vi "adam-analog-outputs.vi"(0 "VISA Refnum in":refnum<visa-resource-name>, 1 "Chassis Settings":T1, 5 "Current AO States":T2, 7 "Analog Outputs in":T2, 9 "chassis-slot":i32, 11 "error in (no error)":errorcluster, 12 "Last cmd":string, 13 "last ack message":string) -> (4 "VISA Refnum out":refnum<visa-resource-name>, 6 "Analog Outputs out":T2, 8 "cmd output":string, 10 "ack message":string, 14 "cmd aknowledged":bool, 15 "error out":errorcluster)   [LabVIEW 2020]
uses:
  controls/analog-output-cluster.ctl
  controls/adam-5000-serial-settings.ctl
panel:
  out "size(s)":i32
  out "loopwise ack":string
  out "OP Num":string
  out "Data":string
  out "live-cmd":string
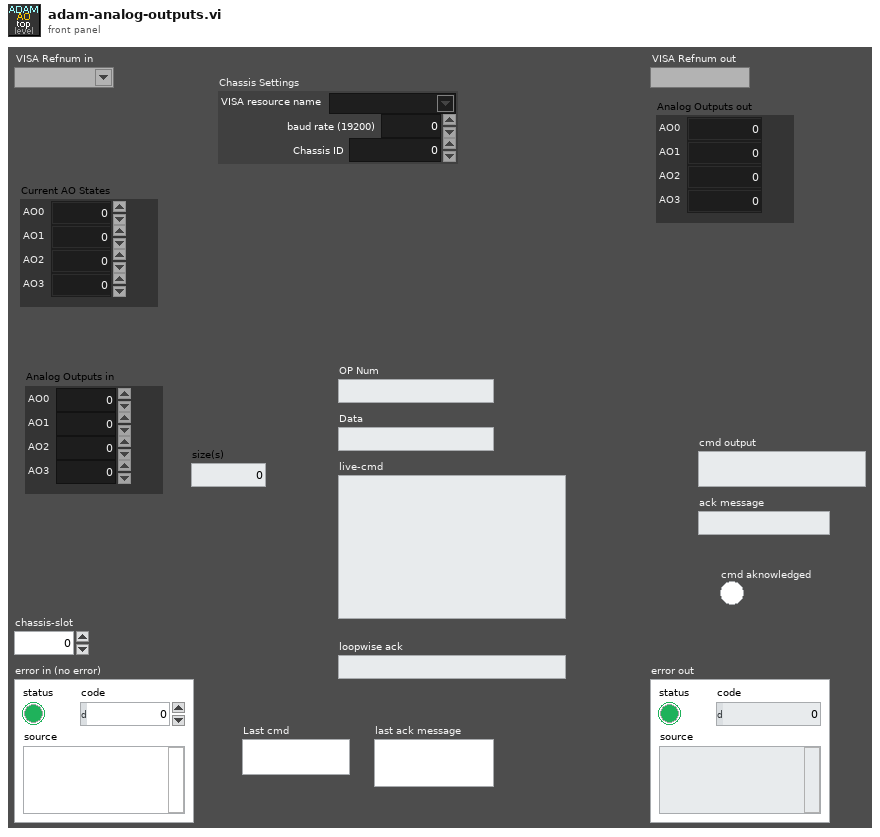
[diagram p1: front panel]
types:
  T1 = typedef "adam-5000-serial-settings.ctl" = cluster{"VISA resource name":refnum<visa-resource-name>, "baud rate (19200)":u32, "Chassis ID":u8}
  T2 = typedef "analog-output-cluster.ctl" = cluster{"AO0":dbl, "AO1":dbl, "AO2":dbl, "AO3":dbl}
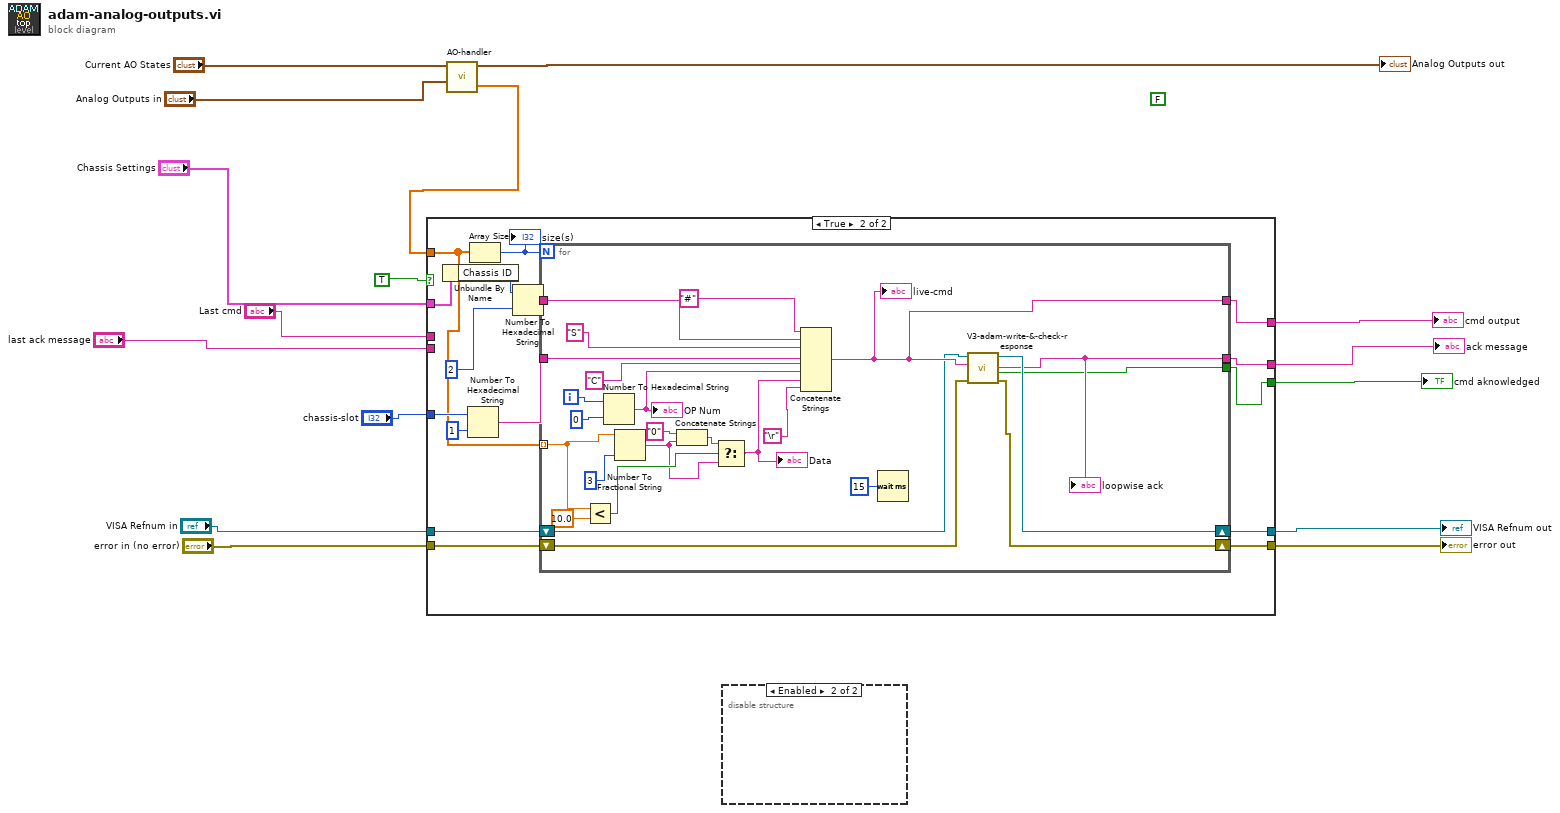
[diagram p0: block diagram]
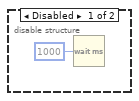
[diagram p2: hidden frame]
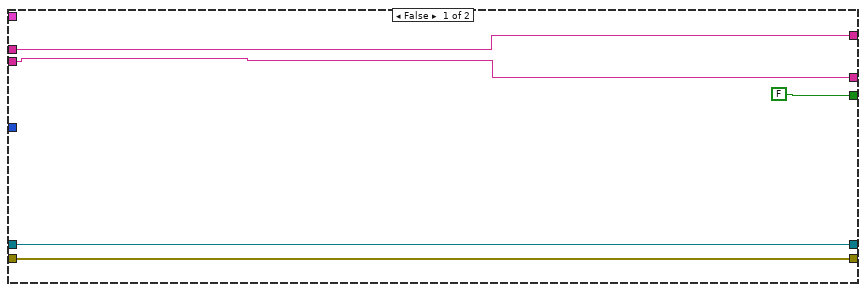
[diagram p3: hidden frame]
diagram:
  (unwired) FALSE ("cmd aknowledged")
  n1 = call "AO-handler.vi"("Analog Outputs Ctrl"="Analog Outputs in", "Analog Output State"="Current AO States") -> ("Analog Outputs"=→"Analog Outputs out":T2, "Analog Val array"=w16:dbl[])  [unwired: 5 in, 3 out]
  n2 = case shown="True" TRUE {
    tunnel: "VISA Refnum in" -> [w21 w33]
    tunnel: "error in (no error)" -> [w19 w32]
    tunnel: [w19 w24] -> w8
    tunnel: [w21 w31] -> w9
    tunnel: [FALSE ("cmd aknowledged") w30] -> w2
    tunnel: [w17 w29] -> w3
    tunnel: [w18 w28] -> w4
    tunnel: "Chassis Settings" -> [_ w27]
    tunnel: "chassis-slot" -> [_ w26]
    tunnel: "Last cmd" -> [w18 _]
    tunnel: "last ack message" -> [w17 _]
    tunnel: w16 -> [_ w25]
    frame False {
    }
    frame True {
      n3 = Unbundle By Name(w27) -> ("Chassis ID"=w37:u8)
      n4 = Number To Hexadecimal String(1:i16 1 ("width (-)"), 2:w26) -> (0:w34:string)
      n5 = Array Size(array=w25) -> (size(s)=w22:i32)
      "size(s)" <- w22
      n6 = Number To Hexadecimal String(1:i16 2 ("width (-)"), 2:w37) -> (0:w23:string)
      n7 = for {
        N: w22 -> [_]
        tunnel: [w45] -> w30
        shift-right: [w47] -> w31
        shift-left: w33 -> [w50]
        shift-right: [w48] -> w24
        shift-left: w32 -> [w49]
        tunnel: w25 -> [w44] mode=indexing
        tunnel: w23 -> [w62]
        tunnel: [w51] -> w28
        tunnel: w34 -> [w60]
        tunnel: [w46] -> w29
        i -> [w58]
        n8 = Less?(x=w44, y=10.0) -> (x < y?=w41:bool)
        n9 = Number To Hexadecimal String(1:i16 0 ("width (-)"), 2:w58) -> (0:w56:string)
        "OP Num" <- w56
        n10 = Number To Fractional String(number=w44, precision (6)=i16 3) -> (F-format string=w39:string)  [unwired: 2 in]
        n11 = Concatenate Strings("0" ("string"), w39) -> (w40:string)
        n12 = Select(t=w40, s=w41, f=w39) -> (s? t:f=w38:string)
        "Data" <- w38
        n13 = Concatenate Strings("#" ("string"), w62, "S" ("string"), w60, "C" ("string"), w56, w38, "\r") -> (w51:string)
        "live-cmd" <- w51
        n14 = Wait (ms)(milliseconds to wait=u32 15) -> ()  [unwired: 1 out]
        n15 = call "V3-adam-write-&-check-response.vi"("error in (no error)"=w49, "write buffer"=w51, "VISA resource name"=w50) -> ("error out"=w48:errorcluster, "cmd aknowledged"=w45:bool, "VISA resource name out"=w47:refnum<visa-resource-name>, "read buffer"=w46:string)  [unwired: 4 in, 1 out]
        "loopwise ack" <- w46
      }
    }
  }
  "VISA Refnum out" <- w9
  "error out" <- w8
  "cmd output" <- w4
  "ack message" <- w3
  "cmd aknowledged" <- w2
  n16 = disable-structure shown="Enabled" {
    frame Disabled {
      n17 = Wait (ms)(milliseconds to wait=u32 1000) -> ()  [unwired: 1 out]
    }
    frame Enabled {
    }
  }
